vi "Send Keyboard Data.vi"(7 "Robot IP":string, 10 "keys pressed":T1(array[ring])) -> ()   [LabVIEW 2015]
uses:
  Common Code/Keyboard Packet.ctl
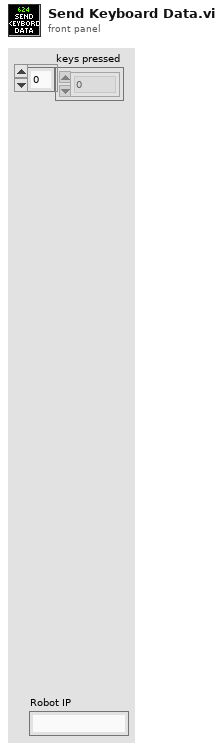
[diagram p1: front panel]
types:
  T1 = enum16{"0", "1", "2", "3", "4", "5", "6", "7", "8", "9", "A", "B", "C", "D", "E", "F", "G", "H", "I", "J", "K", "L", "M", "N", "O", "P", "Q", "R", "S", "T", "U", "V", "W", "X", "Y", "Z", "F1", "F2", "F3", "F4", "F5", "F6", "F7", "F8", "F9", "F10", "F11", "F12", "F13", "F14", "F15", "ADD", "BACK", "BACKSLASH", "CAPITAL", "COMMA", "DECIMAL", "DELETE", "DIVIDE", "DOWN", "END", "EQUALS", "ESCAPE", "GRAVE (`)", "HOME", "INSERT", "LBRACKET", "LCONTROL", "LEFT", "L ALT", "LSHIFT", "LWIN", "MINUS", "MULTIPLY", "NEXT", "NUMLOCK", "NUMPAD_0", "NUMPAD_1", "NUMPAD_2", "NUMPAD_3", "NUMPAD_4", "NUMPAD_5", "NUMPAD_6", "NUMPAD_7", "NUMPAD_8", "NUMPAD_9", "PAUSE", "PERIOD", "PRIOR (PG UP)", "RBRACKET", "RCONTROL", "RETURN", "RIGHT", "R ALT", "RSHIFT", "RWIN", "SCROLL", "SEMICOLON", "SLASH", "SPACE", "SUBTRACT", "TAB", "UP", "ENTER (num pad)", "' (quote)"}[]
  T2 = typedef "Keyboard Packet.ctl" = cluster{"keys pressed":enum16{"0", "1", "2", "3", "4", "5", "6", "7", "8", "9", "A", "B", "C", "D", "E", "F", "G", "H", "I", "J", "K", "L", "M", "N", "O", "P", "Q", "R", "S", "T", "U", "V", "W", "X", "Y", "Z", "F1", "F2", "F3", "F4", "F5", "F6", "F7", "F8", "F9", "F10", "F11", "F12", "F13", "F14", "F15", "ADD", "BACK", "BACKSLASH", "CAPITAL", "COMMA", "DECIMAL", "DELETE", "DIVIDE", "DOWN", "END", "EQUALS", "ESCAPE", "GRAVE (`)", "HOME", "INSERT", "LBRACKET", "LCONTROL", "LEFT", "L ALT", "LSHIFT", "LWIN", "MINUS", "MULTIPLY", "NEXT", "NUMLOCK", "NUMPAD_0", "NUMPAD_1", "NUMPAD_2", "NUMPAD_3", "NUMPAD_4", "NUMPAD_5", "NUMPAD_6", "NUMPAD_7", "NUMPAD_8", "NUMPAD_9", "PAUSE", "PERIOD", "PRIOR (PG UP)", "RBRACKET", "RCONTROL", "RETURN", "RIGHT", "R ALT", "RSHIFT", "RWIN", "SCROLL", "SEMICOLON", "SLASH", "SPACE", "SUBTRACT", "TAB", "UP", "ENTER (num pad)", "' (quote)"}[]}
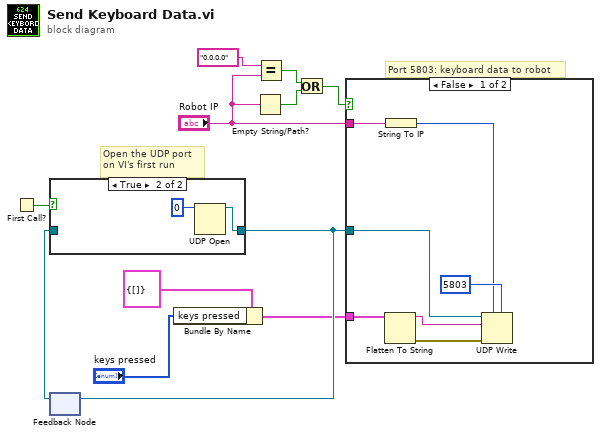
[diagram p0: block diagram]
diagram:
  # "Open the UDP port\non VI's first run"
  # "Port 5803: keyboard data to robot"
  n1 = First Call?() -> (First Call?: T/F=w10:bool)
  n2 = feedback #1() -> (w11:refnum<k16>)  [unwired: 1 in]
  n3 = case shown="True" w10 {
    tunnel: w11 -> [w12 _]
    tunnel: [w12 w13] -> w9
    frame False {
    }
    frame True {
      n4 = UDP Open(11:u16 0 ("port")) -> (port=w13:refnum<k16>)  [unwired: 4 in, 2 out]
    }
  }
  n5 = feedback-in #1(w9) -> ()
  n6 = Bundle By Name(cluster=T2 {"keys pressed"=[]} ("Cluster"), "keys pressed"="keys pressed") -> (w6:T2)
  n7 = Empty String/Path?(string/path="Robot IP") -> (empty?=w2:bool)
  n8 = Equal?(x="0.0.0.0", y="Robot IP") -> (x = y?=w3:bool)
  n9 = Or(x=w3, y=w2) -> (x .or. y?=w1:bool)
  n10 = case shown="False" w1 {
    tunnel: "Robot IP" -> [w19 _]
    tunnel: w9 -> [w20 _]
    tunnel: w6 -> [w18 _]
    frame False {
      n11 = Flatten To String(anything=w18) -> (data string=w17:string, error out=w16:errorcluster)  [unwired: 3 in, 1 out]
      n12 = String To IP(1:w19) -> (0:w15:u32)
      n13 = UDP Write(address=w15, port or service name=u16 5803, connection ID=w20, data in=w17, 8:w16) -> ()  [unwired: 1 in, 2 out]
    }
    frame True {
      # "The robot IP is not\nready yet, don't try\nto send data"
    }
  }
